vi "Write_Wrap_Simple.vi"(4 "Value":T1) -> (1 "Var":refnum<class "Var_U64.lvclass">)   [LabVIEW 2021, in "Var_U64.lvclass"]
uses:
  Var_U64.lvclass
  Type.ctl
  Var_U64.lvclass/Var_U64.ctl
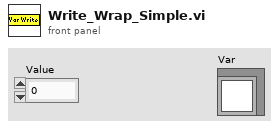
[diagram p1: front panel]
types:
  T1 = typedef "Var_U64.lvclass/Type.ctl" = dbl
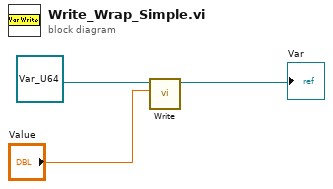
[diagram p0: block diagram]
diagram:
  n1 = call-dynamic "Write.vi"("Value"="Value", "Double Float.lvclass_340760 in"=refnum<class "Var_U64.lvclass"> refnum ("Constants.lvlib:Numeric.lvclass")) -> ("Double Float.lvclass_340760 out"=→"Var":refnum<class "Var_U64.lvclass">)  [unwired: 8 in, 1 out]
